vi "COMP - wavelenght.vi"(11 "COMP-S Andover Filter Wheel":T1) -> (3 "Wavelength (nm)":dbl)   [LabVIEW 2014]
uses:
  Controls/CoMP-S Controls/Emission Line Filter Wheel.ctl
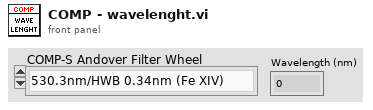
[diagram p1: front panel]
types:
  T1 = typedef "Emission Line Filter Wheel.ctl" = enum16{"530.3nm/HWB 0.34nm (Fe XIV)", "587.6nm/HBW 0.44nm (He I D3)", "637.5nm/HBW 0.53nm (Fe X)", "656.3nm/HBW 0.57nm (H-Alpha)", "789.2nm/HBW 0.85nm (Fe XI)", "854.2nm/HBW 1.01nm (Ca I)", "1074.7nm/HBW 2.34nm (Fe XIII)", "1079.8nm/HBW 1.64nm (Fe XIII)", "1083.0nm/HBW 1.66nm (He I)"}
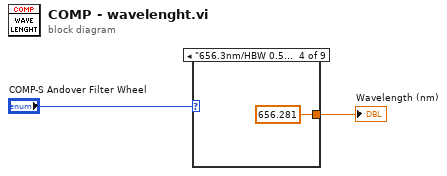
[diagram p0: block diagram]
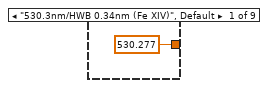
[diagram p2: hidden frame]
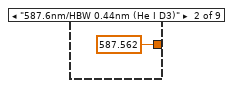
[diagram p3: hidden frame]
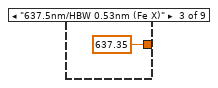
[diagram p4: hidden frame]
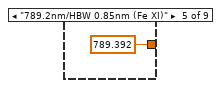
[diagram p5: hidden frame]
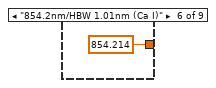
[diagram p6: hidden frame]
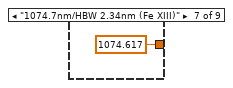
[diagram p7: hidden frame]
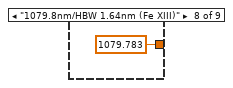
[diagram p8: hidden frame]
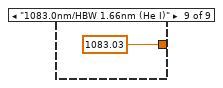
[diagram p9: hidden frame]
diagram:
  n1 = case shown="\"656.3nm/HBW 0.57nm (H-Alpha)\"" "COMP-S Andover Filter Wheel" {
    tunnel: [530.277 ("Wavelength (nm)") 587.562 ("Wavelength (nm)") 637.35 ("Wavelength (nm)") 656.281 ("Wavelength (nm)") 789.392 ("Wavelength (nm)") 854.214 ("Wavelength (nm)") 1074.617 ("Wavelength (nm)") 1079.783 ("Wavelength (nm)") 1083.03 ("Wavelength (nm)")] -> w2
    frame "530.3nm/HWB 0.34nm (Fe XIV)", Default {
    }
    frame "587.6nm/HBW 0.44nm (He I D3)" {
    }
    frame "637.5nm/HBW 0.53nm (Fe X)" {
    }
    frame "656.3nm/HBW 0.57nm (H-Alpha)" {
    }
    frame "789.2nm/HBW 0.85nm (Fe XI)" {
    }
    frame "854.2nm/HBW 1.01nm (Ca I)" {
    }
    frame "1074.7nm/HBW 2.34nm (Fe XIII)" {
    }
    frame "1079.8nm/HBW 1.64nm (Fe XIII)" {
    }
    frame "1083.0nm/HBW 1.66nm (He I)" {
    }
  }
  "Wavelength (nm)" <- w2
